vi "Debug Client Disconnected MHLC.vi"(8 "error in (no error)":errorcluster, 10 "Data in":variant, 11 "AppMgr in":refnum<class "Application Manager.lvclass">) -> (0 "error out":errorcluster, 3 "AppMgr out":refnum<class "Application Manager.lvclass">)   [LabVIEW 2017, in "Application Manager.lvclass"]
doc: "A Debug Client has disconnected from the Debug Server application. Update the corresponding application in the tree with the new information."
uses:
  Application Manager.lvclass
  rqp_Debug Client Disconnected.ctl
  Common VIs/DC_UID.ctl
  Application Manager.lvclass/Application Manager.ctl
  <vilib>/Utility/error.llb/Error Cluster From Error Code.vi
  <vilib>/ErrorRing/Error Ring.xnode
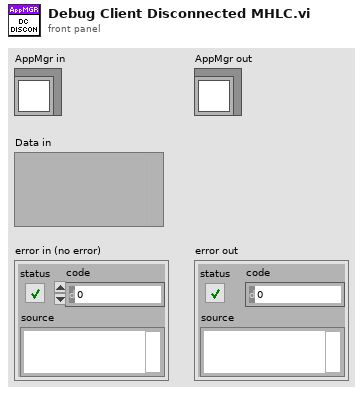
[diagram p1: front panel]
types:
  T1 = typedef "Application Manager.lvclass/rqp_Debug Client Disconnected.ctl" = cluster{"DC_UID":T2}
  T2 = typedef "DC_UID.ctl" = string
  T3 = typedef "Application Manager.lvclass/Debug Client Data.ctl" = cluster{"DC_UID":T2, "IP Address":string, "Worker Data":T4[], "Connected":bool}
  T4 = typedef "Application Manager.lvclass/Worker Data.ctl" = cluster{"ID":string, "VI Ref":refnum<vi>, "VI Path":path, "CloneID":string, "Type":T5, "Worker Status":string}
  T5 = typedef "Workers.lvlib/Worker.lvclass/Worker Type.ctl" = enum16{"SL", "DL"}
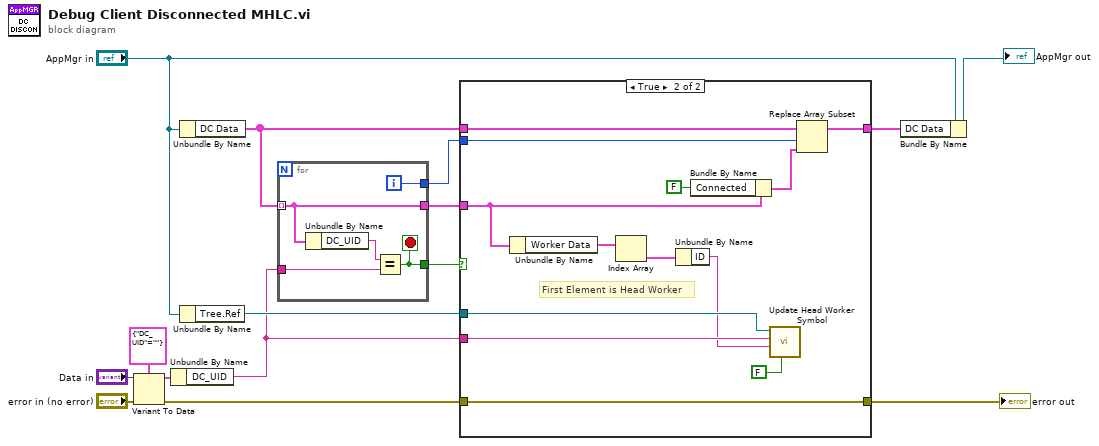
[diagram p0: block diagram]
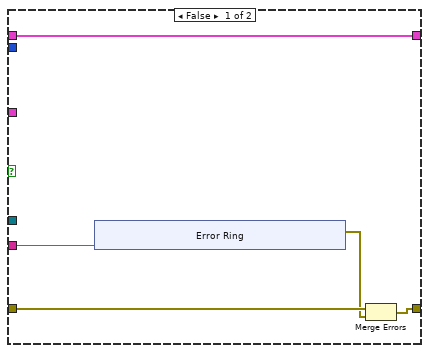
[diagram p2: hidden frame]
diagram:
  n1 = Variant To Data(error in="error in (no error)", type=T1 {"DC_UID"=""} ("Data"), Variant="Data in") -> (data=w9:T1, error out=w12:errorcluster)
  n2 = Unbundle By Name(w9) -> ("DC_UID"=w11:T2)
  n3 = Unbundle By Name("AppMgr in") -> ("DC Data"=w2:T3[])
  n4 = Unbundle By Name("AppMgr in") -> ("Tree.Ref"=w15:refnum<vi>)
  n5 = for {
    tunnel: w2 -> [w17] mode=indexing
    tunnel: w11 -> [w19]
    tunnel: [w18] -> w10
    tunnel: [w17] -> w14
    tunnel: [w16] -> w1
    i -> [w16]
    stop <- w18 stop-if-true
    n6 = Unbundle By Name(w17) -> ("DC_UID"=w20:T2)
    n7 = Equal?(x=w20, y=w19) -> (x = y?=w18:bool)
  }
  n8 = case shown="True" w10 {
    tunnel: w11 -> [w25 w42]
    tunnel: w12 -> [w24 w40]
    tunnel: [w23 w40] -> w13
    tunnel: w14 -> [_ w35]
    tunnel: w15 -> [_ w43]
    tunnel: [w21 w38] -> w3
    tunnel: w2 -> [w21 w39]
    tunnel: w1 -> [_ w37]
    frame False {
      n9 = xnode "Error Ring"("parameter 0"=w25) -> ("error out"=w22:errorcluster)
      n10 = Merge Errors(w24, w22) -> (w23:errorcluster)
    }
    frame True {
      # "First Element is Head Worker"
      n11 = Unbundle By Name(w35) -> ("Worker Data"=w36:T4[])
      n12 = Index Array(array=w36) -> (element=w45:T4)  [unwired: 1 in]
      n13 = Unbundle By Name(w45) -> ("ID"=w41:string)
      n14 = Bundle By Name(cluster=w35, "Connected"=FALSE) -> (w34:T3)
      n15 = call "Update Head Worker Symbol.vi"("Connected?"=FALSE, "WID"=w41, "DC_UID"=w42, "Tree Ref"=w43) -> ()  [unwired: 7 in, 1 out]
      n16 = Replace Array Subset(array=w39, new element=w34, index=w37) -> (w38:T3[])
    }
  }
  "error out" <- w13
  n17 = Bundle By Name(cluster="AppMgr in", "DC Data"=w3) -> (→"AppMgr out":refnum<class "Application Manager.lvclass">)
